vi "LEBITplc.Bob1toBunSetValue.vi"(0 "i ref in":refnum<vi>, 1 "Nickname in":string, 2 "i attribute in":T1, 3 "index in":i32, 4 "value":dbl, 5 "error in":errorcluster) -> (13 "In Range?":bool, 14 "i ref out":refnum<vi>, 15 "Nicknames out":string[](array[string]), 16 "Index out":i32[](array[numeric]), 17 "values":dbl[](array[numeric]), 18 "Log Out?":bool[](array[boolean]), 19 "error out":errorcluster)   [LabVIEW 2014, in "LEBITplc.lvlib"]
uses:
  LEBITplc.lvlib
  LEBITplc.i attribute.ctl
panel:
  in  "file path (dialog if empty)":path=path "\\\\Projects\\proj1/lebit/Data Exchange/data/IonGuideControl/Conversion/MassConversion.txt"
  out "i attribute out":T1
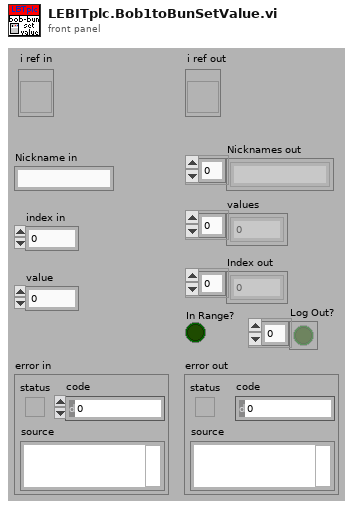
[diagram p1: front panel]
types:
  T1 = typedef "LEBITplc.lvlib/LEBITplc.i attribute.ctl" = cluster{"LLFLocation":string, "SetFileLocation":string, "nickNames":string[], "setValuePLCServiceID":i32[], "GUIServiceID":i32[], "monValuePLC":string[], "SetValueServiceID":i32[], "MonValueServiceID":i32[], "SetValue":dbl[][], "SetValueMin":dbl[], "SetValueMax":dbl[], "SetValueInfoServiceID":i32[], "GUINames":string[], "ListOfBases":string[], "Scale":dbl[], "Offset":dbl[], "setValuePLC":string[], "BaseName":string[], "ScaleServiceID":i32[], "OffsetServiceID":i32[], "AllPLCValues":string[], "CondSpecialArray":string[][], "CondSpecialIndex":i32[], "CondSpecialMonValue":dbl[], "RecentlyChanged":i32[], "SetFileLocationID":i32, "Dependent-Monitors":string[][], "LastLoadedFiles":string[], "IonGuideCalibLocation":string, "Monitor Dependent":string[], "Special":string[], "PLC?":bool[], "Start Date":string, "ListOfBasesServiceID":i32, "SETRA VISA resource":refnum<visa-resource-name>}
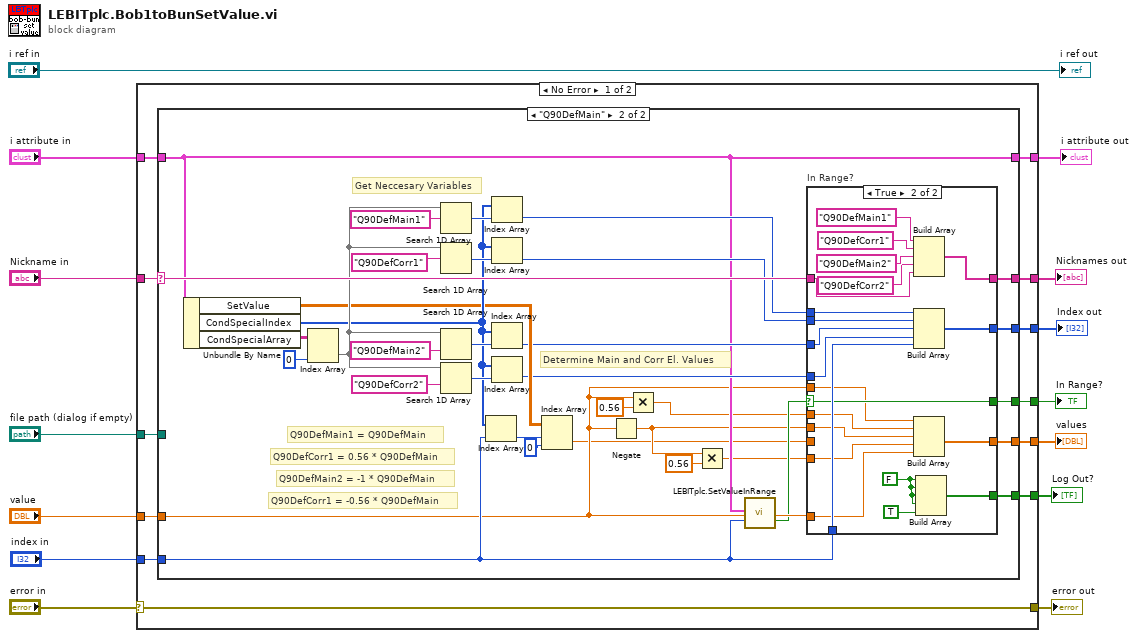
[diagram p0: block diagram]
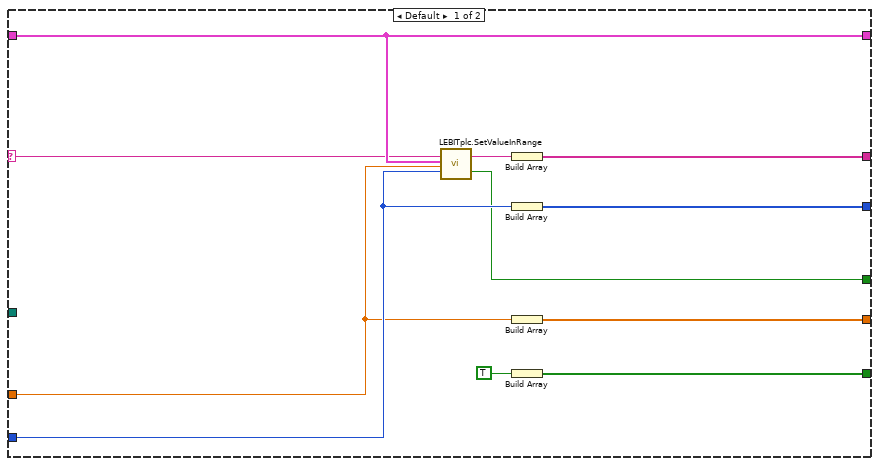
[diagram p2: hidden frame]
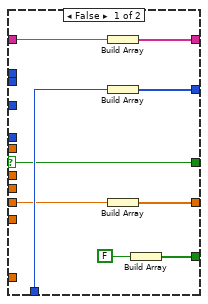
[diagram p3: hidden frame]
diagram:
  n1 = case shown="No Error" "error in" {
    selector: "error in" -> [w16 w105]
    tunnel: "Nickname in" -> [w26 _]
    tunnel: "i attribute in" -> [w25 w106]
    tunnel: [w24 w106] -> w12
    tunnel: "value" -> [w23 _]
    tunnel: [w22 _] -> w10
    tunnel: [w21 _] -> w9
    tunnel: "file path (dialog if empty)" -> [w20 _]
    tunnel: "index in" -> [w19 _]
    tunnel: [w18 _] -> w6
    tunnel: [w17 _] -> w5
    tunnel: [w16 w105] -> w3
    tunnel: [w15 _] -> w1
    frame No Error {
      n2 = case shown="\"Q90DefMain\"" w26 {
        selector: w26 -> [w33 w69]
        tunnel: w25 -> [w34 w48]
        tunnel: [w34 w48] -> w24
        tunnel: w23 -> [w29 w40]
        tunnel: [w37 w70] -> w22
        tunnel: [w36 w68] -> w21
        tunnel: w20 -> [_ _]
        tunnel: w19 -> [w31 w51]
        tunnel: [w35 w57] -> w18
        tunnel: [w30 w45] -> w17
        tunnel: [w27 w39] -> w15
        frame Default {
          n3 = call "LEBITplc.SetValueInRange.vi"("CommandName in"=w33, "i attribute in"=w34, "value in"=w29, "index of element"=w31) -> ("CommandName out"=w32:string, "In Range?"=w30:bool)  [unwired: 11 in, 3 out]
          n4 = Build Array(w32) -> (w36:string[])
          n5 = Build Array(w31) -> (w35:i32[])
          n6 = Build Array(w29) -> (w37:dbl[])
          n7 = Build Array(TRUE) -> (w27:bool[])
        }
        frame "Q90DefMain" {
          # "Q90DefCorr1 = -0.56 * Q90DefMain"
          # "Q90DefMain2 = -1 * Q90DefMain"
          # "Q90DefCorr1 = 0.56 * Q90DefMain"
          # "Q90DefMain1 = Q90DefMain"
          # "Determine Main and Corr El. Values"
          # "Get Neccesary Variables"
          n8 = Unbundle By Name(w48) -> ("SetValue"=w53:dbl[][], "CondSpecialIndex"=w58:i32[], "CondSpecialArray"=w67:string[][])
          n9 = Index Array(array=w67, index (col)=0 ("index (row)")) -> (element=w59:string[])  [unwired: 1 in]
          n10 = Search 1D Array(1D array=w59, element="Q90DefMain1") -> (index of element=w61:i32)  [unwired: 1 in]
          n11 = Search 1D Array(1D array=w59, element="Q90DefCorr1") -> (index of element=w63:i32)  [unwired: 1 in]
          n12 = Search 1D Array(1D array=w59, element="Q90DefMain2") -> (index of element=w66:i32)  [unwired: 1 in]
          n13 = Search 1D Array(1D array=w59, element="Q90DefCorr2") -> (index of element=w65:i32)  [unwired: 1 in]
          n14 = Index Array(array=w58, index=w51) -> (element=w64:i32)
          n15 = Index Array(array=w58, index=w61) -> (element=w56:i32)
          n16 = Index Array(array=w58, index=w63) -> (element=w55:i32)
          n17 = Index Array(array=w58, index=w66) -> (element=w52:i32)
          n18 = Index Array(array=w58, index=w65) -> (element=w49:i32)
          n19 = Index Array(array=w53, index (row)=w64, index (col)=0 ("disabled index (col)")) -> (element=w38:dbl)
          n20 = Negate(x=w40) -> (-x=w41:dbl)
          n21 = Multiply(x=w40, y=0.56 ("ratio")) -> (x*y=w43:dbl)
          n22 = Multiply(x=w41, y=0.56 ("ratio")) -> (x*y=w42:dbl)
          n23 = call "LEBITplc.SetValueInRange.vi"("i attribute in"=w48, "value in"=w40, "index of element"=w51) -> ("value out"=w50:dbl, "In Range?"=w44:bool)  [unwired: 12 in, 3 out]
          n24 = case "In Range?" shown="True" w44 {
            selector: w44 -> [w78 w90]
            tunnel: [w77 w104] -> w70
            tunnel: w69 -> [w81 w91]
            tunnel: [w82 w101] -> w68
            tunnel: [w80 w100] -> w57
            tunnel: w56 -> [_ w99]
            tunnel: w55 -> [_ w98]
            tunnel: w51 -> [w79 w95]
            tunnel: w52 -> [_ w97]
            tunnel: w50 -> [_ w94]
            tunnel: w49 -> [_ w96]
            tunnel: [w78 w90] -> w45
            tunnel: w43 -> [_ w88]
            tunnel: w40 -> [_ w89]
            tunnel: w41 -> [_ w87]
            tunnel: w42 -> [_ w86]
            tunnel: [w75 w85] -> w39
            tunnel: w38 -> [w74 _]
            frame False {
              n25 = Build Array(w81) -> (w82:string[])
              n26 = Build Array(w79) -> (w80:i32[])
              n27 = Build Array(w74) -> (w77:dbl[])
              n28 = Build Array(FALSE) -> (w75:bool[])
            }
            frame True {
              w83 = FALSE
              n29 = Build Array("Q90DefMain1" ("element"), "Q90DefCorr1" ("element"), "Q90DefMain2" ("element"), "Q90DefCorr2" ("element"), w91) -> (w101:string[])
              n30 = Build Array(w99, w98, w97, w96, w95) -> (w100:i32[])
              n31 = Build Array(w89, w88, w87, w86, w94) -> (w104:dbl[])
              n32 = Build Array(w83, w83, w83, w83, TRUE) -> (w85:bool[])
            }
          }
        }
      }
    }
    frame Error {
    }
  }
  "i attribute out" <- w12
  "values" <- w10
  "Nicknames out" <- w9
  "Index out" <- w6
  "In Range?" <- w5
  "error out" <- w3
  "Log Out?" <- w1
  "i ref out" <- "i ref in"
